vi "OpenVIReferenceExperiment.vi"() -> ()   [LabVIEW 2020]
panel:
  out "error out":errorcluster
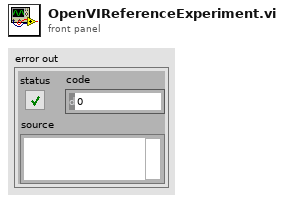
[diagram p1: front panel]
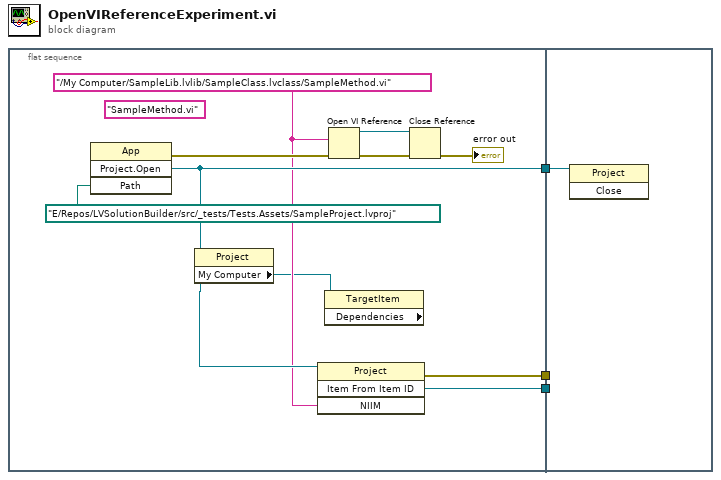
[diagram p0: block diagram]
diagram:
  n1 = flat-sequence {
    tunnel: [w8] -> w3
    tunnel: [w7] -> w2
    tunnel: [w6] -> w1
    tunnel: w3 -> [w14]
    tunnel: w2 -> [_]
    tunnel: w1 -> [_]
    frame #0 {
      w5 = "/My Computer/SampleLib.lvlib/SampleClass.lvclass/SampleMethod.vi"
      (unwired) "SampleMethod.vi"
      n2 = invoke class="App" method="Project.Open"("Path"=path "E:/Repos/LVSolutionBuilder/src/_tests/Tests.Assets/SampleProject.lvproj") -> (error out=w10:errorcluster, "Project:Open"=w8:refnum<vi>)  [unwired: 3 in, 2 out]
      n3 = property class="Project"(reference=w8) -> ("My Computer"=w4:refnum<vi>)  [unwired: 1 in, 2 out]
      n4 = invoke class="Project" method="Item From Item ID"(reference=w8, "NIIM"=w5) -> (error out=w6:errorcluster, "GetItemFromNIIM"=w7:refnum<vi>)  [unwired: 2 in, 2 out]
      n5 = property class="TargetItem" props=["Dependencies"](reference=w4) -> ()  [unwired: 1 in, 3 out]
      n6 = Open VI Reference(vi path=w5, error in (no error)=w10) -> (vi reference=w13:refnum<vi>, error out=w12:errorcluster)  [unwired: 4 in]
      n7 = Close Reference(reference=w13, error in (no error)=w12) -> (error out=→"error out":errorcluster)
    }
    frame #1 {
      n8 = invoke class="Project" method="Close"(reference=w14) -> ()  [unwired: 2 in, 3 out]
    }
  }
